vi "Get Protocol Type.vi"(8 "error in (no error)":errorcluster, 11 "protocol in":refnum<class "Protocol Parent.lvclass">) -> (0 "error out":errorcluster, 2 "protocol type":T1=enum."AK RS-XXX", 3 "protocol out":refnum<class "Protocol Parent.lvclass">)   [LabVIEW 2023, in "Protocols.lvlib" / "Protocol Parent.lvclass"]
doc: "Returns a protocol type Enum matching the protocol wired to the Protocol Parent in terminal.\n\nInput:\nProtocol Parent in: represents an instance of the Protocol Parent class and any other class which inherits it.\n\nOutput: \nProtocol Parent out: represents an instance of the Protocol Parent class provided as input.\nProtocol Type: represents the type of the protocol in Enum format."
uses:
  Protocol Parent.lvclass
  Types/Protocol Type.ctl
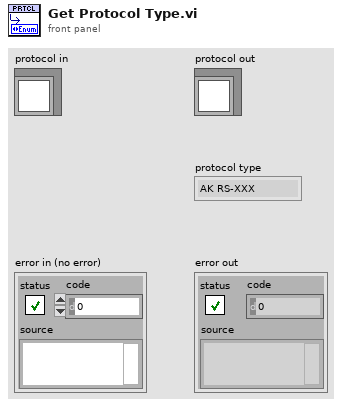
[diagram p1: front panel]
types:
  T1 = typedef "Protocols.lvlib/Protocol Parent.lvclass/Protocol Type.ctl" = enum16{"RS-XXX", "AK RS-XXX", "VISA", "TCPIP", "AK TCPIP", "UDP", "GPIB ConvBox"}
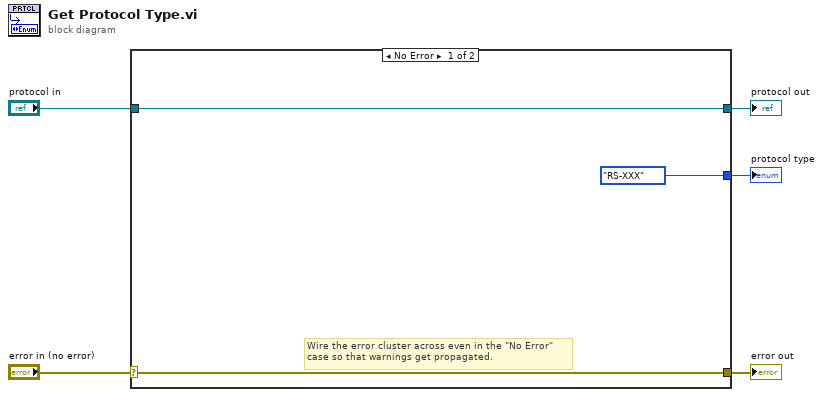
[diagram p0: block diagram]
diagram:
  n1 = case shown="No Error" "error in (no error)" {
    selector: "error in (no error)" -> [w7 w10]
    tunnel: [w7 w10] -> w4
    tunnel: [w8 w9] -> w2
    tunnel: "protocol in" -> [w8 w9]
    tunnel: [Protocol_Type."RS-XXX" ("Protocol out") _] -> w1
    frame No Error {
      # "Wire the error cluster across even in the \"No Error\"\ncase so that warnings get propagated."
    }
    frame Error {
    }
  }
  "error out" <- w4
  "protocol out" <- w2
  "protocol type" <- w1
